vi "数据补传对话框.vi"(11 "起始时间":timestamp) -> (0 "参数数值out":T1={"CODMn"=TRUE, "CODCr"=TRUE, "DO"=TRUE, "铜"=TRUE, "PH"=TRUE, "氨氮"=TRUE, "比电导率"=TRUE, "水温"=TRUE, "COD"=TRUE, "浊度"=TRUE, "总氮"=TRUE, "总磷"=TRUE, "叶绿素a"=TRUE, "藻密度"=TRUE, "水位"=TRUE, "流速"=TRUE, "瞬时流量"=TRUE, "累积流量"=TRUE, "亚硝氮"=TRUE, "硫化物"=TRUE, "ORP"=TRUE, "铅"=TRUE, "镉"=TRUE, "锌"=TRUE, "镍"=TRUE, "锰"=TRUE, "汞"=TRUE, "气温"=TRUE, "气压"=TRUE, "风速"=TRUE, "风向"=TRUE, "盐度"=TRUE, "磷酸盐"=TRUE, "硝氮"=TRUE, "氟化物"=TRUE, "挥发酚"=TRUE, "氯化物"=TRUE}, 1 "结束时间输出":timestamp, 2 "起始时间输出":timestamp, 3 "输出":bool=TRUE, 5 "只补小时数据输出":bool)   [LabVIEW 2016, in "数据传输系统-02.lvlib"]
panel:
  in  "只补小时数据":bool
  in  "补传参数":bool
  in  "结束时间":timestamp
  in  "取消":bool
  in  "确定":bool
  # "数据补传时间选择"
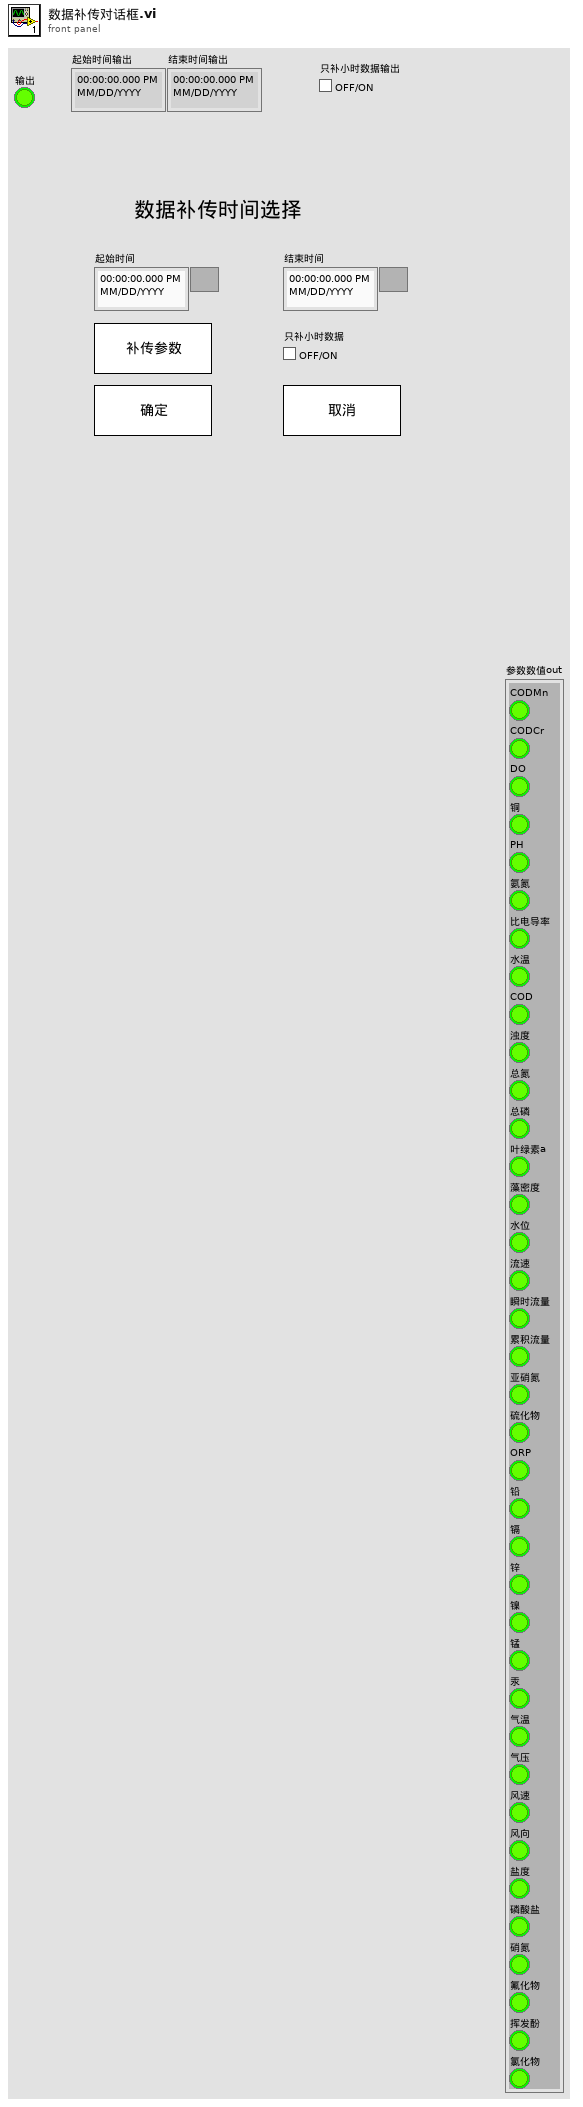
[diagram p1: front panel]
types:
  T1 = cluster{"CODMn":bool, "CODCr":bool, "DO":bool, "铜":bool, "PH":bool, "氨氮":bool, "比电导率":bool, "水温":bool, "COD":bool, "浊度":bool, "总氮":bool, "总磷":bool, "叶绿素a":bool, "藻密度":bool, "水位":bool, "流速":bool, "瞬时流量":bool, "累积流量":bool, "亚硝氮":bool, "硫化物":bool, "ORP":bool, "铅":bool, "镉":bool, "锌":bool, "镍":bool, "锰":bool, "汞":bool, "气温":bool, "气压":bool, "风速":bool, "风向":bool, "盐度":bool, "磷酸盐":bool, "硝氮":bool, "氟化物":bool, "挥发酚":bool, "氯化物":bool}
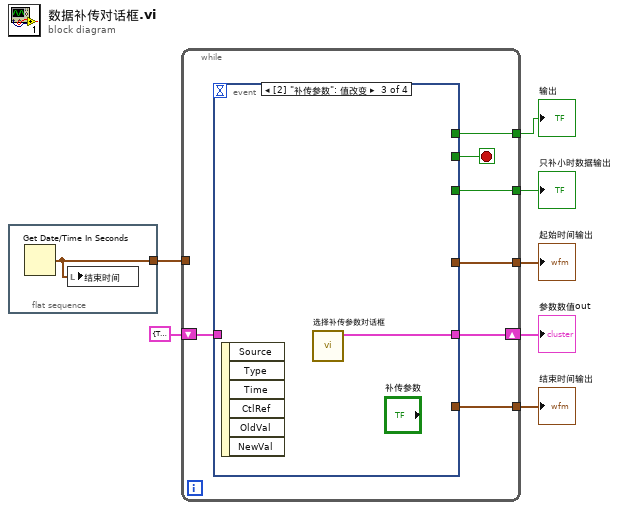
[diagram p0: block diagram]
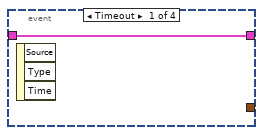
[diagram p2: hidden frame]
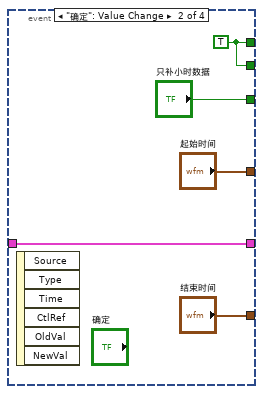
[diagram p3: hidden frame]
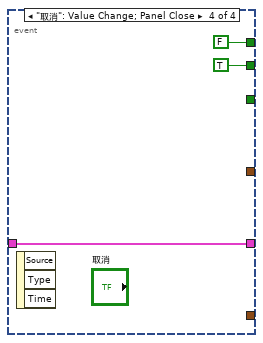
[diagram p4: hidden frame]
diagram:
  n1 = flat-sequence {
    tunnel: [w8] -> w4
    frame #0 {
      n2 = Get Date/Time In Seconds() -> (seconds since 1Jan1904=w8:timestamp)
      n3 = local write "结束时间"(w8) -> ()
    }
  }
  n4 = while {
    tunnel: [w15] -> w7
    tunnel: [w13] -> w6
    tunnel: [w12] -> w5
    tunnel: w4 -> [_]
    shift-right: [w11] -> w3
    shift-left: T1 {"CODMn"=TRUE, "CODCr"=TRUE, "DO"=TRUE, "铜"=TRUE, "PH"=TRUE, "氨氮"=TRUE, "比电导率"=TRUE, "水温"=TRUE, "COD"=TRUE, "浊度"=TRUE, "总氮"=TRUE, "总磷"=TRUE, "叶绿素a"=TRUE, "藻密度"=TRUE, "水位"=TRUE, "流速"=TRUE, "瞬时流量"=TRUE, "累积流量"=TRUE, "亚硝氮"=TRUE, "硫化物"=TRUE, "ORP"=TRUE, "铅"=TRUE, "镉"=TRUE, "锌"=TRUE, "镍"=TRUE, "锰"=TRUE, "汞"=TRUE, "气温"=TRUE, "气压"=TRUE, "风速"=TRUE, "风向"=TRUE, "盐度"=TRUE, "磷酸盐"=TRUE, "硝氮"=TRUE, "氟化物"=TRUE, "挥发酚"=TRUE, "氯化物"=TRUE} ("参数数值out") -> [w10]
    tunnel: [w9] -> w1
    stop <- w14 stop-if-true
    n5 = event shown="[2] \"补传参数\": 值改变" {
      selector: _ -> [_ _ _ _]
      dyn-events: _ -> [_ _ _ _]
      timeout: _ -> [_ _ _ _]
      tunnel: [_ w21 _ FALSE] -> w15
      tunnel: [_ w21 _ TRUE] -> w14
      tunnel: [_ "起始时间" _ _] -> w13
      tunnel: [_ "结束时间" _ _] -> w12
      tunnel: [w16 w18 w22 w23] -> w11
      tunnel: w10 -> [w16 w18 _ w23]
      tunnel: [_ "只补小时数据" _ _] -> w9
      event Timeout {
        n6 = event-data() -> ()  [unwired: 1 in, 3 out]
      }
      event "确定": Value Change {
        w21 = TRUE
        n7 = event-data() -> ()  [unwired: 1 in, 6 out]
      }
      event "补传参数": Value Change {
        n8 = event-data() -> ()  [unwired: 1 in, 6 out]
        n9 = call "选择补传参数对话框.vi"() -> ("参数数值out"=w22:T1)  [unwired: 11 in]
      }
      event "取消": Value Change; Panel Close {
        n10 = event-data() -> ()  [unwired: 1 in, 3 out]
      }
    }
  }
  "输出" <- w7
  "起始时间输出" <- w6
  "结束时间输出" <- w5
  "参数数值out" <- w3
  "只补小时数据输出" <- w1
